vi "Date and Time.vi"() -> (0 "Time string.":string, 1 "Date string.":string)   [LabVIEW 2010]
panel:
  # "No inputs."
  # "Outputs:"
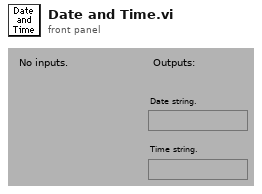
[diagram p1: front panel]
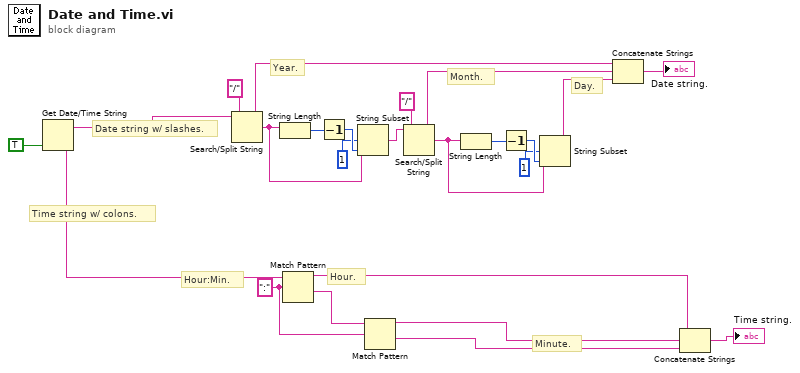
[diagram p0: block diagram]
diagram:
  w3 = ":" ("search string/char (-)")
  # "Hour."
  # "Minute."
  # "Hour:Min."
  # "Day."
  # "Month."
  # "Year."
  # "Time string w/ colons."
  # "Date string w/ slashes."
  n1 = Get Date/Time String(want seconds? (F)=TRUE) -> (date string=w9:string, time string=w6:string)  [unwired: 2 out]
  n2 = Search/Split String(string=w9, search string/char (-)="/") -> (substring before match=w11:string, match + rest of string=w20:string)  [unwired: 2 out]
  n3 = String Length(string=w20) -> (length=w23:i32)
  n4 = Match Pattern(string=w6, regular expression=w3) -> (before substring=w5:string, after substring=w4:string)  [unwired: 3 out]
  n5 = Decrement(x=w23) -> (x-1=w22:i32)
  n6 = String Subset(string=w20, offset (0)=1, length (rest)=w22) -> (substring=w14:string)
  n7 = Match Pattern(string=w4, regular expression=w3) -> (before substring=w2:string, after substring=w1:string)  [unwired: 3 out]
  n8 = Search/Split String(string=w14, search string/char (-)="/") -> (substring before match=w12:string, match + rest of string=w15:string)  [unwired: 2 out]
  n9 = String Length(string=w15) -> (length=w18:i32)
  n10 = Decrement(x=w18) -> (x-1=w17:i32)
  n11 = String Subset(string=w15, offset (0)=1, length (rest)=w17) -> (substring=w13:string)
  n12 = Concatenate Strings(w11, w12, w13) -> (→"Date string.":string)
  n13 = Concatenate Strings(w5, w2, w1) -> (→"Time string.":string)
